vi "Flush Output.vi"(8 "error in (no error)":errorcluster, 11 "CLI in":refnum<class "CLI.lvclass">) -> (0 "error out":errorcluster, 3 "CLI out":refnum<class "CLI.lvclass">)   [LabVIEW 2017, in "CLI.lvclass"]
doc: "Flushes the stdout and stderr streams manually.\n\nThis is required for more advanced interfaces where you don't use new lines. If you write with line endings the console will be flushed there anyway."
uses:
  CLI.lvclass
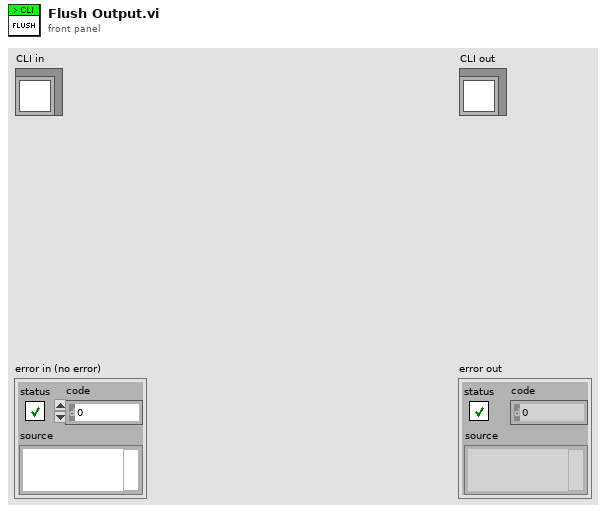
[diagram p1: front panel]
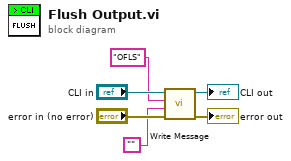
[diagram p0: block diagram]
diagram:
  n1 = call "Write Message.vi"("error in (no error)"="error in (no error)", "Message Contents"="", "Message Type"="OFLS", "CLI in"="CLI in") -> ("error out"=→"error out":errorcluster, "CLI out"=→"CLI out":refnum<class "CLI.lvclass">)  [unwired: 6 in]
